vi "allstar.vi"() -> ()   [LabVIEW 2018]
panel:
  out "left":dbl
  out "error out":errorcluster
  in  "error in (no error)":errorcluster
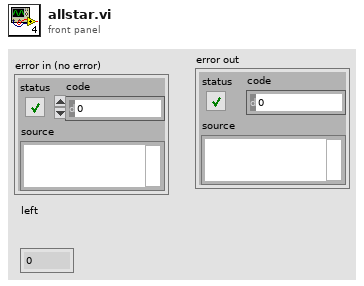
[diagram p1: front panel]
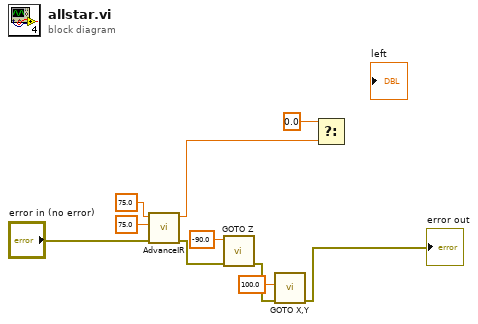
[diagram p0: block diagram]
diagram:
  n1 = call "AdvanceIR.vi"("error in (no error)"="error in (no error)", "side"=75.0, "straight"=75.0) -> ("error out"=w7:errorcluster, "誤差"=w2:dbl)  [unwired: 6 in, 1 out]
  n2 = call "GOTO Z.vi"("error in (no error)"=w7, "Z"=-90.0) -> ("error out"=w5:errorcluster)  [unwired: 9 in]
  n3 = call "GOTO X,Y.vi"("error in (no error)"=w5, "Y"=100.0) -> ("error out"=→"error out":errorcluster)  [unwired: 9 in]
  n4 = Select(t=0.0, f=w2) -> ()  [unwired: 1 in, 1 out]
